vi "Write Get Data.vi"(8 "error in (no error)":errorcluster, 10 "Get Data":bool, 11 "Start DAC in":refnum<class "Start DAC.lvclass">) -> (0 "error out":errorcluster, 3 "Start DAC out":refnum<class "Start DAC.lvclass">)   [LabVIEW 2019, in "DAC Process.lvlib" / "Start DAC.lvclass"]
uses:
  Start DAC.lvclass
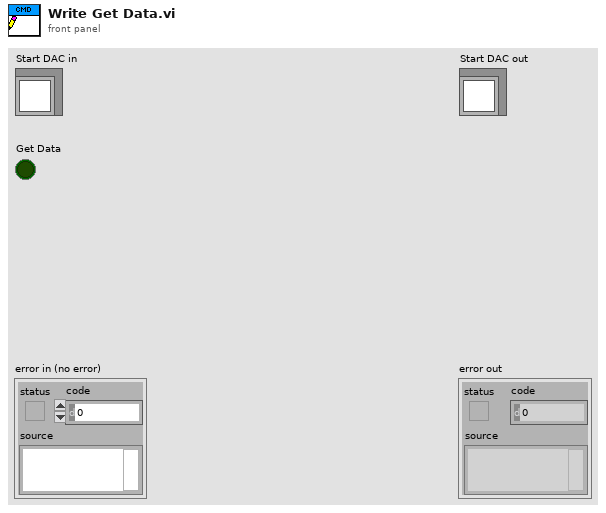
[diagram p1: front panel]
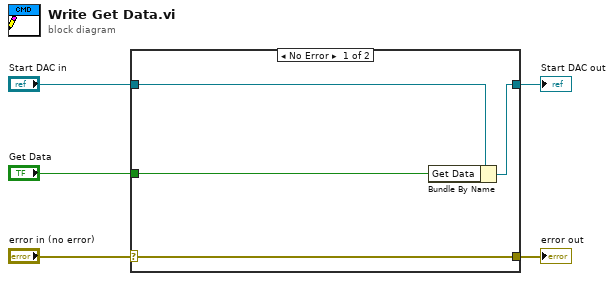
[diagram p0: block diagram]
diagram:
  n1 = case shown="No Error" "error in (no error)" {
    selector: "error in (no error)" -> [w9 w10]
    tunnel: [w9 w10] -> w4
    tunnel: [w7 w11] -> w2
    tunnel: "Start DAC in" -> [w8 w11]
    tunnel: "Get Data" -> [w6 _]
    frame No Error {
      n2 = Bundle By Name(cluster=w8, "Get Data"=w6) -> (w7:refnum<class "Start DAC.lvclass">)
    }
    frame Error {
    }
  }
  "error out" <- w4
  "Start DAC out" <- w2
